vi "joystick to desired height.vi"(8 "CurrentHeight":dbl, 11 "Joystick Input":dbl) -> (3 "Desired Height":dbl)   [LabVIEW 2015]
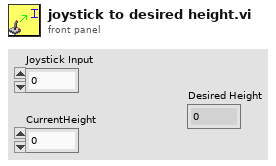
[diagram p1: front panel]
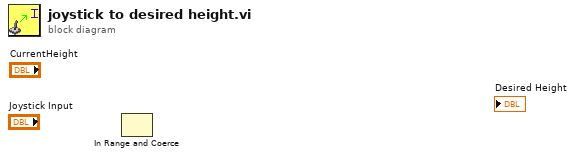
[diagram p0: block diagram]
diagram:
  n1 = In Range and Coerce() -> ()  [unwired: 3 in, 2 out]
